vi "CRYSearch Matrix Element.vi"(8 "start index":i32, 9 "element":i32, 10 "index (row)":i32, 11 "matrix in":i32[][](array[numeric])) -> (3 "index of element":i32)   [LabVIEW 2013]
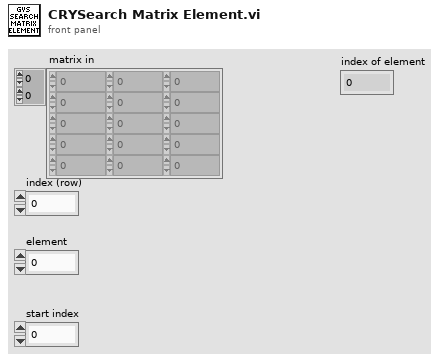
[diagram p1: front panel]
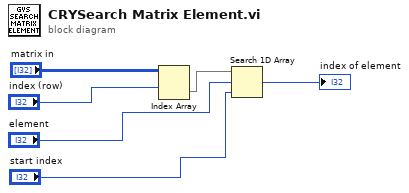
[diagram p0: block diagram]
diagram:
  n1 = Index Array(array="matrix in", index (row)="index (row)") -> (element=w6:i32[])  [unwired: 1 in]
  n2 = Search 1D Array(1D array=w6, element="element", start index (0)="start index") -> (index of element=→"index of element":i32)
